vi "practica9b.vi"() -> ()   [LabVIEW 2013]
panel:
  out "URL 2":string
  in  "URL":string
  in  "stop":bool
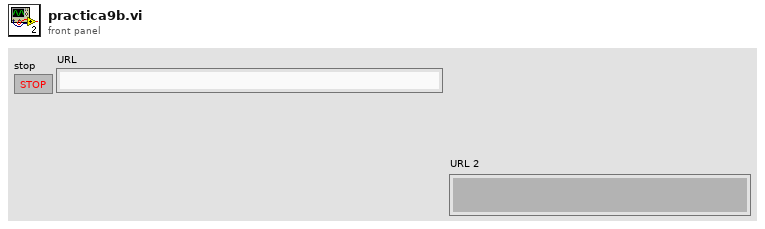
[diagram p1: front panel]
types:
  T1 = enum16{"Read", "Write", "ReadWrite", "BufferedRead", "BufferedReadWrite"}
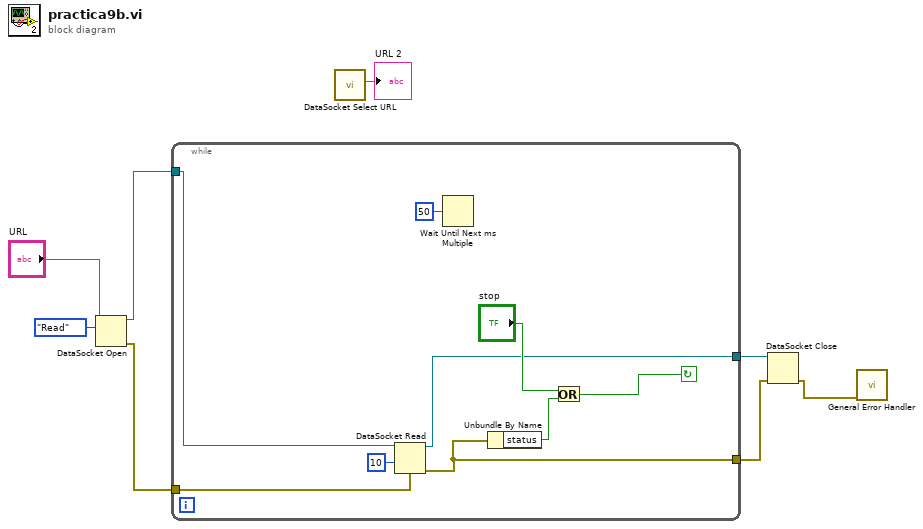
[diagram p0: block diagram]
diagram:
  n1 = DataSocket Open(10:T1."Read" ("mode"), 11:"URL") -> (0:w8:errorcluster, 3:w7:refnum<k13>)  [unwired: 2 in]
  n2 = while {
    tunnel: w8 -> [w13]
    tunnel: w7 -> [w11]
    tunnel: [w12] -> w6
    tunnel: [w9] -> w2
    stop <- w14 continue-if-true
    n3 = DataSocket Read(8:w13, 9:10 ("ms timeout (10000)"), 11:w11) -> (0:w12:errorcluster, 3:w9:refnum<k13>)  [unwired: 2 in, 5 out]
    n4 = Wait Until Next ms Multiple(millisecond multiple=u32 50) -> ()  [unwired: 1 out]
    n5 = Unbundle By Name(w12) -> ("status"=w15:bool)
    n6 = Or(x="stop", y=w15) -> (x .or. y?=w14:bool)
  }
  n7 = call <vilib>:"DataSocket Select URL.vi"() -> ("URL"=→"URL 2":string)  [unwired: 9 in, 2 out]
  n8 = DataSocket Close(8:w6, 11:w2) -> (0:w5:errorcluster)  [unwired: 1 in, 1 out]
  n9 = call <vilib>:"General Error Handler.vi"("error in (no error)"=w5) -> ()  [unwired: 10 in, 5 out]
